vi "Identify Instrument Type.vi"(11 "Resource Name in":refnum<k15>) -> (2 "Resource Type":T1, 3 "Resource Name out":refnum<k15>)   [LabVIEW 2023]
uses:
  DC Ins Type.ctl
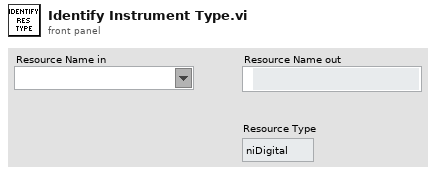
[diagram p1: front panel]
types:
  T1 = typedef "DC Ins Type.ctl" = enum16{"niDigital", "niDCPower", "undefined"}
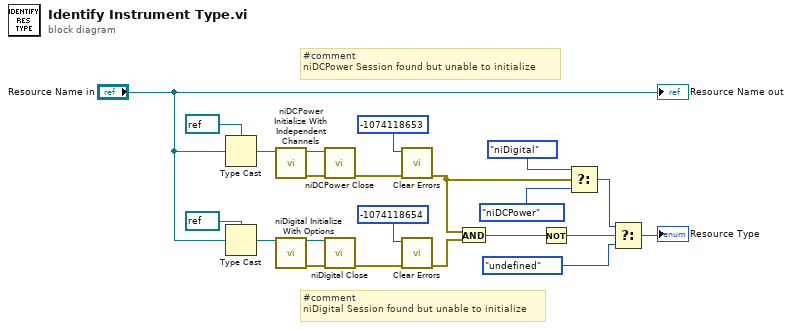
[diagram p0: block diagram]
diagram:
  # "#comment\nniDigital Session found but unable to initialize"
  # "#comment\nniDCPower Session found but unable to initialize"
  n1 = Type Cast(type=refnum<k15> refnum ("reference"), x="Resource Name in") -> (*(type *) &x=w6:refnum<k15>)
  n2 = Type Cast(type=refnum<k15> refnum ("reference"), x="Resource Name in") -> (*(type *) &x=w18:refnum<k15>)
  n3 = call <instrlib>:"niDCPower Initialize With Independent Channels.vi"("resource name"=w6) -> ("error out"=w19:errorcluster, "instrument handle out"=w20:refnum<k15>)  [unwired: 9 in]
  n4 = call <instrlib>:"niDigital Initialize With Options.vi"("resource name"=w18) -> ("instrument handle"=w17:refnum<k15>, "error out"=w16:errorcluster)  [unwired: 13 in]
  n5 = call <instrlib>:"niDCPower Close.vi"("error in (no error)"=w19, "instrument handle"=w20) -> ("error out"=w14:errorcluster)  [unwired: 9 in]
  n6 = call <instrlib>:"niDigital Close.vi"("instrument handle"=w17, "error in"=w16) -> ("error out"=w2:errorcluster)  [unwired: 13 in]
  n7 = call <vilib>:"Clear Errors.vi"("error in (no error)"=w14, "specific error code to clear (0: all)"=-1074118653) -> ("error out"=w5:errorcluster)  [unwired: 4 in, 1 out]
  n8 = call <vilib>:"Clear Errors.vi"("error in (no error)"=w2, "specific error code to clear (0: all)"=-1074118654) -> ("error out"=w1:errorcluster)  [unwired: 4 in, 1 out]
  n9 = And(x=w5, y=w1) -> (x .and. y?=w13:bool)
  n10 = Not(x=w13) -> (.not. x?=w11:bool)
  n11 = Select(t=DC_Ins_Type."niDigital" ("Resource Type"), s=w5, f=DC_Ins_Type."niDCPower" ("Resource Type")) -> (s? t:f=w15:T1)
  n12 = Select(t=w15, s=w11, f=DC_Ins_Type."undefined" ("Resource Type")) -> (s? t:f=→"Resource Type":T1)
  "Resource Name out" <- "Resource Name in"
